vi "反应性模拟计算.vi"(0 "循环次数":bool, 1 "λi*Ci(0)":sgl[][](array[numeric])=[[82.89727, 82.892685, 82.89905, 82.885956]], 3 "N(0)IN":sgl[](array[numeric]), 5 "βi":sgl[](array[numeric])=[0.000176, 0.001258, 0.001139, 0.002309, 0.000791, 0.000288], 7 "λi":sgl[](array[numeric])=[0.0125, 0.0306, 0.1167, 0.3133, 1.217, 3.266], 9 "中子寿命":sgl=2.3e-05, 11 "源项":sgl, 12 "采集间隔":sgl=0.05, 13 "中子注量率":sgl[][](array[numeric])=[[82.89727, 82.892685, 82.89905, 82.885956]]) -> (2 "λi*Ci(t)":sgl[][](array[numeric]), 8 "反应性OUT":sgl[][](array[numeric]), 14 "N(0)OUT":sgl[](array[numeric]))   [LabVIEW 2020]
uses:
  <vilib>/Analysis/baseanly.llb/Mean (DBL).vi
  <vilib>/express/express arith-compare/Formula/XNode/ExpressFormulaBlockNode.xnode
  <vilib>/Analysis/NI_AALBase.lvlib
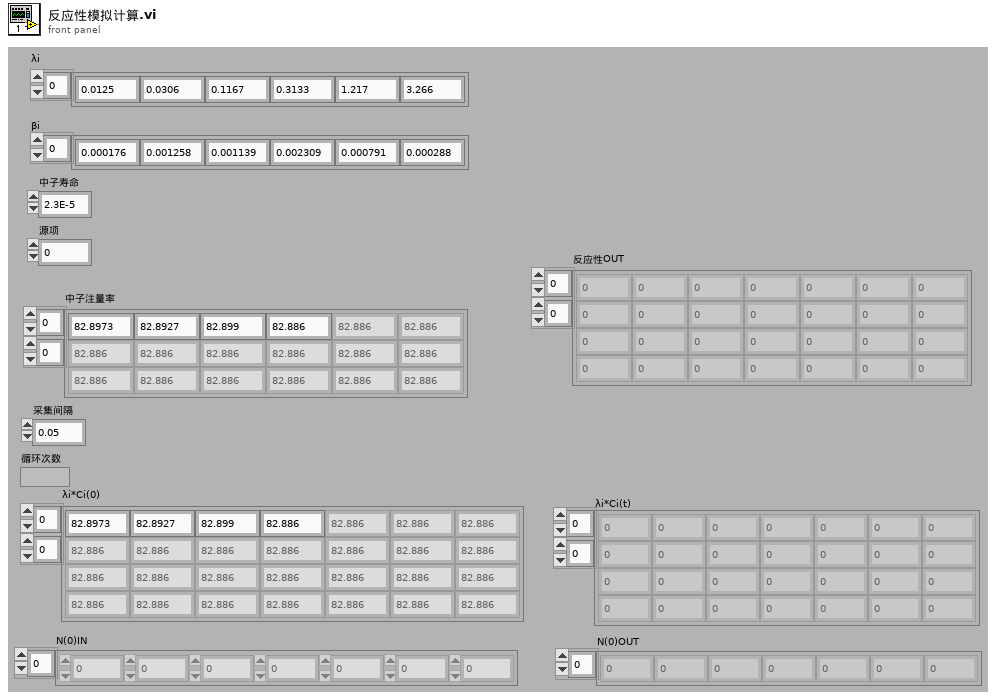
[diagram p1: front panel]
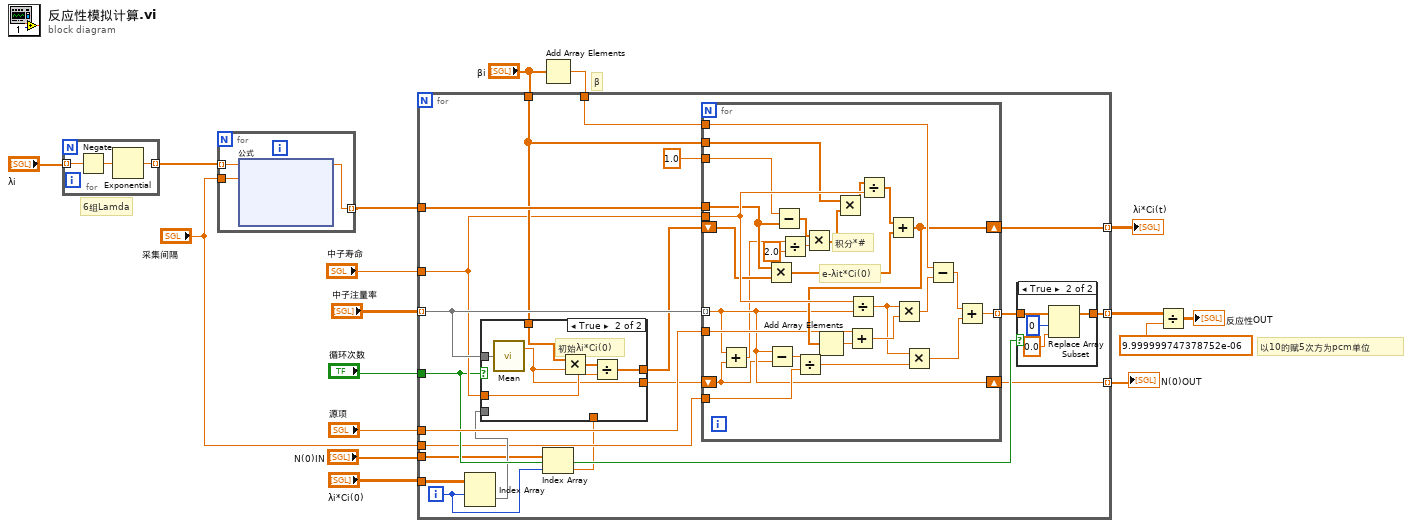
[diagram p0: block diagram]
diagram:
  # "6组Lamda"
  # "β"
  # "以10的赋5次方为pcm单位"
  n1 = for {
    tunnel: [w20] -> w3 mode=indexing
    tunnel: "λi" -> [w19] mode=indexing
    n2 = Negate(x=w19) -> (-x=w18:sgl)
    n3 = Exponential(1:w18) -> (0:w20:sgl)
  }
  n4 = for {
    tunnel: "采集间隔" -> [w22]
    tunnel: [w21] -> w2 mode=indexing
    tunnel: w3 -> [w23] mode=indexing
    n5 = xnode "公式"("X1"=w23, "X2"=w22) -> ("结果"=w21:sgl)  [unwired: 1 in, 1 out]
  }
  n6 = Add Array Elements(numeric array="βi") -> (sum=w9:sgl)
  n7 = for {
    tunnel: w9 -> [w53]
    tunnel: [w43] -> w16 mode=indexing
    tunnel: w2 -> [w52]
    tunnel: "中子注量率" -> [w50] mode=indexing
    tunnel: "βi" -> [w49]
    tunnel: "源项" -> [w47]
    tunnel: "中子寿命" -> [w48]
    tunnel: "λi*Ci(0)" -> [w41]
    tunnel: [w46] -> w13 mode=indexing
    tunnel: "循环次数" -> [w45]
    tunnel: "采集间隔" -> [w39]
    tunnel: [w38] -> w5 mode=indexing
    tunnel: "N(0)IN" -> [w37]
    i -> [w36]
    n8 = Index Array(array=w41, index (row)=w36) -> (element=w40:sgl[])  [unwired: 1 in]
    n9 = Index Array(array=w37, index=w36) -> (element=w35:sgl)
    n10 = case shown="True" w45 {
      tunnel: w50 -> [_ w62]
      tunnel: w49 -> [_ w66]
      tunnel: [w60 w65] -> w42
      tunnel: w48 -> [_ w64]
      tunnel: w40 -> [w60 _]
      tunnel: [w59 w61] -> w34
      tunnel: w35 -> [w59 _]
      frame False {
        # "后续Ci(0)"
      }
      frame True {
        # "初始λi*Ci(0)"
        n11 = call-poly <vilib>:"Mean.vi"("X"=w62) -> ("mean"=w61:dbl)  [unwired: 1 out]
        n12 = Multiply(x=w66, y=w61) -> (x*y=w63:dbl[])
        n13 = Divide(x=w63, y=w64) -> (x/y=w65:dbl[])
      }
    }
    n14 = for {
      tunnel: w50 -> [w71] mode=indexing
      tunnel: w53 -> [w92]
      tunnel: w47 -> [w72]
      shift-right: [w83] -> w46
      shift-left: w42 -> [w84]
      tunnel: w48 -> [w91]
      tunnel: [w81] -> w44 mode=indexing
      tunnel: w52 -> [w76]
      tunnel: sgl 1.0 -> [w75]
      tunnel: w49 -> [w90]
      shift-right: [w71] -> w38
      shift-left: w34 -> [w70]
      tunnel: w39 -> [w78]
      # "积分*#"
      # "e-λit*Ci(0)"
      n15 = Add(x=w71, y=w70) -> (x+y=w69:dbl)
      n16 = Multiply(x=w76, y=w84) -> (x*y=w85:dbl[])
      n17 = Subtract(x=w71, y=w70) -> (x-y=w74:dbl)
      n18 = Subtract(x=w75, y=w76) -> (x-y=w88:sgl[])
      n19 = Divide(x=w69, y=sgl 2.0) -> (x/y=w67:dbl)
      n20 = Divide(x=w74, y=w78) -> (x/y=w77:dbl)
      n21 = Multiply(x=w88, y=w67) -> (x*y=w73:dbl[])
      n22 = Multiply(x=w90, y=w73) -> (x*y=w87:dbl[])
      n23 = Divide(x=w91, y=w71) -> (x/y=w80:sgl)
      n24 = Divide(x=w87, y=w91) -> (x/y=w86:dbl[])
      n25 = Add(x=w86, y=w85) -> (x+y=w83:dbl[])
      n26 = Add Array Elements(numeric array=w83) -> (sum=w89:dbl)
      n27 = Add(x=w72, y=w89) -> (x+y=w94:dbl)
      n28 = Multiply(x=w80, y=w94) -> (x*y=w93:dbl)
      n29 = Multiply(x=w80, y=w77) -> (x*y=w79:dbl)
      n30 = Subtract(x=w92, y=w93) -> (x-y=w82:dbl)
      n31 = Add(x=w82, y=w79) -> (x+y=w81:dbl)
    }
    n32 = case shown="True" w45 {
      tunnel: w44 -> [w54 w58]
      tunnel: [w54 w56] -> w43
      frame False {
      }
      frame True {
        n33 = Replace Array Subset(array=w58, new element=sgl 0.0 ("新元素/子数组"), index=0) -> (w56:dbl[])
      }
    }
  }
  "λi*Ci(t)" <- w13
  "N(0)OUT" <- w5
  n34 = Divide(x=w16, y=sgl 1e-05) -> (x/y=→"反应性OUT":dbl[][])
